vi "Module Loop.vi"(8 "error in (no error)":errorcluster, 11 "Telemetry Command Module in":refnum<class "Telemetry Command Module.lvclass">) -> (0 "error out":errorcluster, 3 "Telemetry Command Module out":refnum<class "Telemetry Command Module.lvclass">)   [LabVIEW 2020, in "VolatusGUI.lvlib" / "Telemetry Command Module.lvclass"]
uses:
  Telemetry Command Module.lvclass
  C:/dev/lv20CE/relink/lv-volatus/Volatus/Module/Module.lvclass
  Volatus/Module/Module.lvclass/Module.ctl
  Volatus/Module/Module.lvclass
  Volatus/MessageQ/MessageQ.lvclass/MessageQ.ctl
  Channel Selection.ctl
  <vilib>/Utility/error.llb/Error Cluster From Error Code.vi
  Telemetry Command Module.lvclass/Telemetry Command Module.ctl
  Volatus/MessageQ/MessageQ.lvclass
panel:
  in  "Clear Filter":bool
  in  "Filter":string
  in  "Tree":string(tree)
  out "error out 2":errorcluster
  out "Resource":string
  out "Group":string
  out "Task":string
  out "Channel":string
  out "Node":string
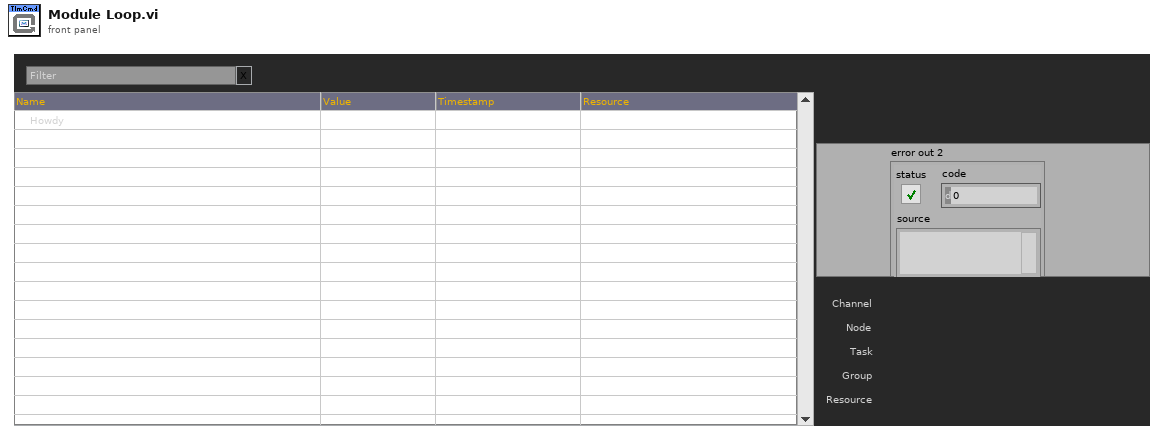
[diagram p1: front panel]
types:
  T1 = typedef "imagedata.ctl" = cluster{"image type":i32, "image depth":i32, "image":u8[], "mask":u8[], "colors":u32[], "Rectangle":cluster{"left":i16, "top":i16, "right":i16, "bottom":i16}}
  T2 = enum32{"Invalid", "Standard", "Closed", "Hidden", "Minimized", "Maximized"}
  T3 = typedef "VolatusGUI.lvlib/Telemetry Command Module.lvclass/Channel Selection.ctl" = cluster{"Node":string, "Group":string, "Channel":string}
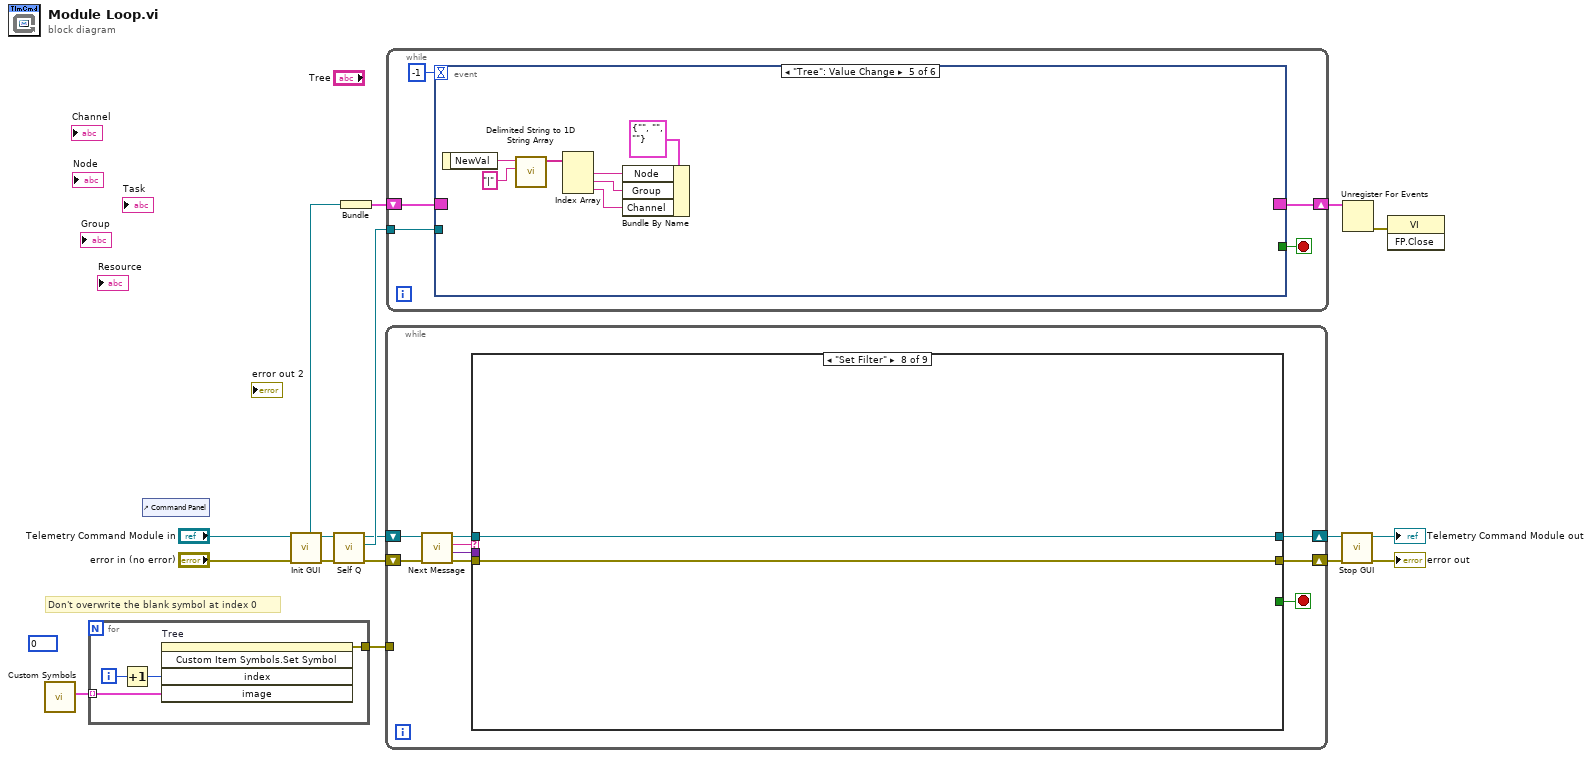
[diagram p0: block diagram]
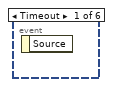
[diagram p2: hidden frame]
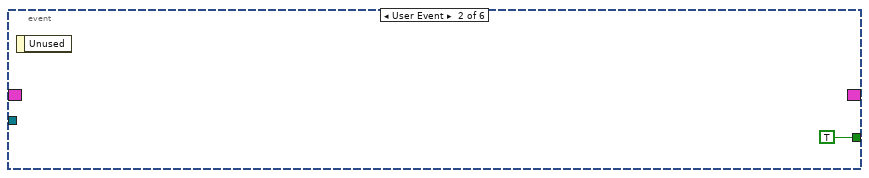
[diagram p3: hidden frame]
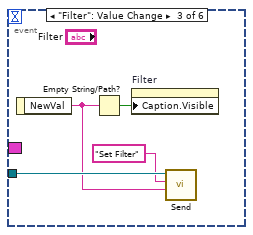
[diagram p4: hidden frame]
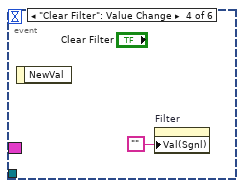
[diagram p5: hidden frame]
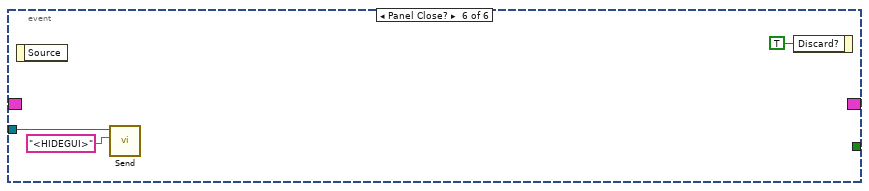
[diagram p6: hidden frame]
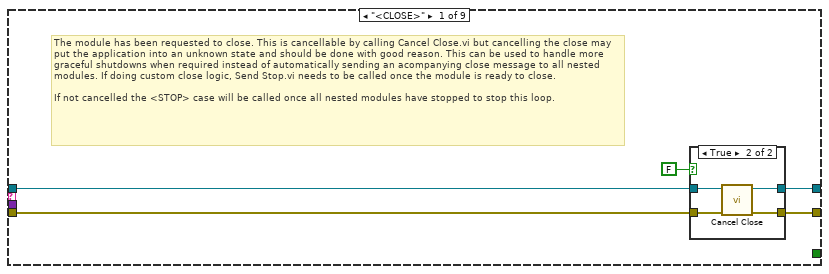
[diagram p7: hidden frame]
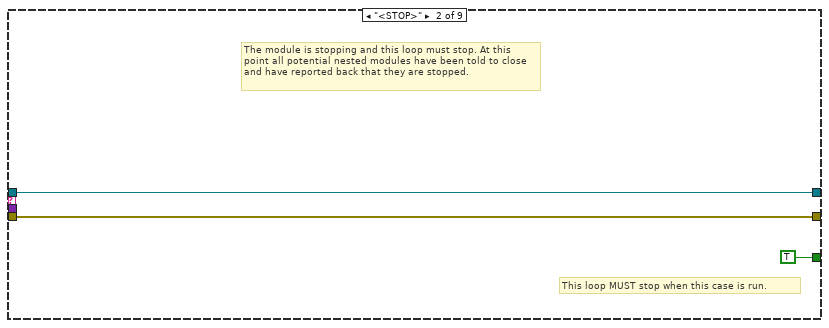
[diagram p9: hidden frame]
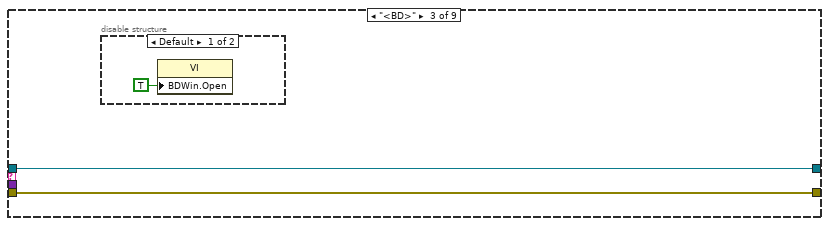
[diagram p10: hidden frame]
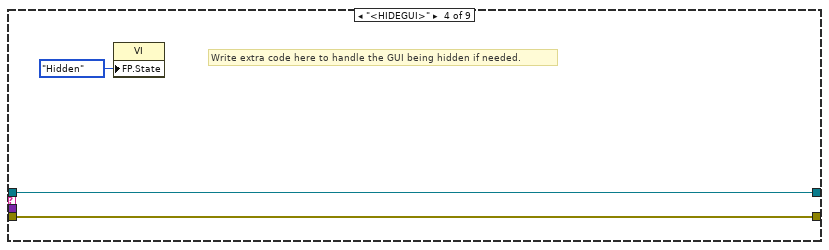
[diagram p12: hidden frame]
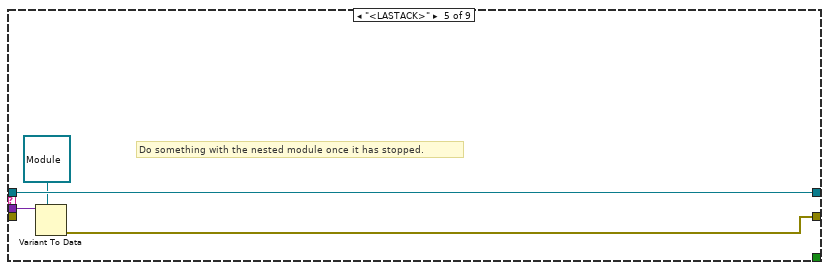
[diagram p13: hidden frame]
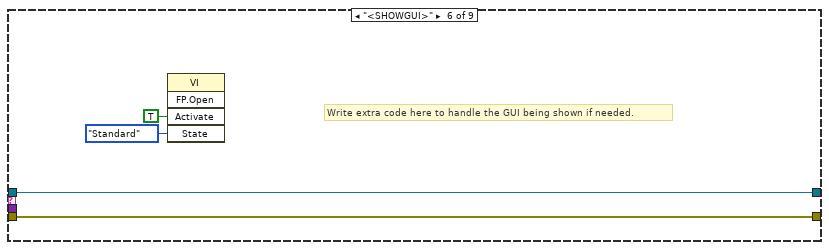
[diagram p14: hidden frame]
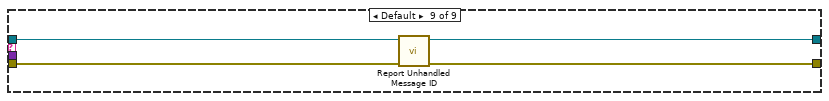
[diagram p16: hidden frame]
diagram:
  (unwired) 0
  # "Don't overwrite the blank symbol at index 0"
  n1 = call "Custom Symbols.vi"() -> ("Custom symbols"=w2:T1[])  [unwired: 11 in]
  n2 = for {
    tunnel: w2 -> [w17] mode=indexing
    tunnel: [w16] -> w1
    i -> [w19]
    n3 = Increment(x=w19) -> (x+1=w18:i32)
    n4 = invoke on="Tree" class="Tree (strict)" method="Custom Item Symbols.Set Symbol"("index"=w18, "image"=w17) -> (error out=w16:errorcluster)  [unwired: 3 in, 4 out]
  }
  n5 = control-ref of="Command Panel"() -> ()  [unwired: 1 out]
  n6 = call "Init GUI.vi"("Module in"="Telemetry Command Module in") -> ("Module out"=w9:refnum<class "Telemetry Command Module.lvclass">, "Event Reg"=w14:refnum<event-registration>)  [unwired: 9 in]
  n7 = call "Self Q.vi"("Module in"=w9) -> ("Self Q"=w8:refnum<class "MessageQ.lvclass">, "Module out"=w7:refnum<class "Telemetry Command Module.lvclass">)  [unwired: 9 in]
  n8 = Bundle("Event Reg"=w14) -> (w10:cluster{"Event Reg":refnum<event-registration>})  [unwired: 1 in]
  n9 = while {
    shift-right: [w23] -> w12
    shift-left: w7 -> [w28]
    shift-right: [w22] -> w13
    shift-left: "error in (no error)" -> [w27]
    tunnel: w1 -> [_]
    stop <- w21 stop-if-true
    n10 = call "Next Message.vi"("error in (no error)"=w27, "Module in"=w28) -> ("error out"=w26:errorcluster, "Data"=w20:variant, "ID"=w25:string, "Module out"=w24:refnum<class "Telemetry Command Module.lvclass">)  [unwired: 6 in]
    n11 = case shown="\"Set Filter\"" w25 {
      tunnel: w26 -> [w31 w41 w43 w47 _ w55 w57 w59 w64]
      tunnel: w24 -> [w32 w42 w44 w48 w52 w56 w58 w60 w62]
      tunnel: [w30 w42 w44 w48 w52 w56 w58 w60 w61] -> w23
      tunnel: [w29 w41 w43 w47 w49 w55 w57 w59 w63] -> w22
      tunnel: [_ TRUE _ _ _ _ _ _ _] -> w21
      tunnel: w20 -> [_ _ _ _ w51 _ _ _ _]
      frame "<CLOSE>" {
        # "The module has been requested to close. This is cancellable by calling Cancel Close.vi but cancelling the close may put the application into an unknown state and should be done with good reason. This can be used to handle more graceful shutdowns when required instead of automatically sending an acompanying close message to all nested modules. If doing custom close logic, Send Stop.vi needs to be called once the module is ready to close.\n\nIf not cancelled the <STOP> case will be called once all nested modules have stopped to stop this loop."
        n12 = case shown="True" FALSE {
          tunnel: w31 -> [w34 w39]
          tunnel: [w34 w38] -> w29
          tunnel: w32 -> [w35 w37]
          tunnel: [w35 w36] -> w30
          frame False {
          }
          frame True {
            n13 = call "Cancel Close.vi"("error in (no error)"=w39, "Module in"=w37) -> ("error out"=w38:errorcluster, "Module out"=w36:refnum<class "Telemetry Command Module.lvclass">)  [unwired: 8 in]
          }
        }
      }
      frame "<STOP>" {
        # "This loop MUST stop when this case is run."
        # "The module is stopping and this loop must stop. At this point all potential nested modules have been told to close and have reported back that they are stopped."
      }
      frame "<BD>" {
        n14 = disable-structure shown="Default" {
          frame condition #0 (active) {
            n15 = property class="VI"("BDWin.Open"=TRUE ("Block Diagram Window:Open")) -> ()  [unwired: 2 in, 2 out]
          }
          frame condition #1 {
          }
        }
      }
      frame "<HIDEGUI>" {
        # "Write extra code here to handle the GUI being hidden if needed."
        n16 = property class="VI"("FP.State"=T2."Hidden" ("Front Panel Window:State")) -> ()  [unwired: 2 in, 2 out]
      }
      frame "<LASTACK>" {
        # "Do something with the nested module once it has stopped."
        n17 = Variant To Data(type=refnum<class "Module.lvclass"> refnum ("Volatus:Module"), Variant=w51) -> (error out=w49:errorcluster)  [unwired: 1 in, 1 out]
      }
      frame "<SHOWGUI>" {
        # "Write extra code here to handle the GUI being shown if needed."
        n18 = invoke class="VI" method="FP.Open"("Activate"=TRUE ("Activate?"), "State"=T2."Standard") -> ()  [unwired: 3 in, 5 out]
      }
      frame "<TIMEOUT>" {
        # "No message for this module was received in time"
      }
      frame "Set Filter" {
      }
      frame Default {
        n19 = call "Report Unhandled Message ID.vi"("error in (no error)"=w64, "Module in"=w62) -> ("error out"=w63:errorcluster, "Module out"=w61:refnum<class "Telemetry Command Module.lvclass">)  [unwired: 8 in]
      }
    }
  }
  n20 = while {
    tunnel: w8 -> [w69]
    shift-right: [w67] -> w11
    shift-left: w10 -> [w68]
    stop <- w66 stop-if-true
    n21 = event shown="[4] \"Tree\": Value Change" {
      selector: w68 -> [_ _ _ _ _ _]
      dyn-events: [_ _ _ _ _ _] -> w67
      timeout: -1 -> [_ _ _ _ _ _]
      tunnel: w69 -> [_ _ w74 _ _ w84]
      tunnel: [_ TRUE _ _ _ _] -> w66
      event Timeout {
        n22 = event-data() -> ()  [unwired: 1 in, 1 out]
      }
      event User Event {
        n23 = event-data() -> ()  [unwired: 1 in, 1 out]
      }
      event "Filter": Value Change {
        n24 = event-data() -> ("NewVal"=w73:string)  [unwired: 1 in]
        n25 = Empty String/Path?(string/path=w73) -> (empty?=w71:bool)
        n26 = property on="Filter" class="Str"("Caption.Visible"=w71) -> ()  [unwired: 2 in, 2 out]
        n27 = call "Send.vi"("Data"=w73, "ID"="Set Filter", "MessageQ in"=w74) -> ()  [unwired: 7 in, 2 out]
      }
      event "Clear Filter": Value Change {
        n28 = event-data() -> ()  [unwired: 1 in, 1 out]
        n29 = property on="Filter" class="Str"("Val(Sgnl)"="") -> ()  [unwired: 2 in, 2 out]
      }
      event "Tree": Value Change {
        n30 = event-data() -> ("NewVal"=w82:string)  [unwired: 1 in]
        n31 = call <vilib>:"Delimited String to 1D String Array.vi"("delimiter"="|", "delimited string"=w82) -> ("string array"=w80:string[])  [unwired: 9 in]
        n32 = Index Array(array=w80) -> (element #1=w78:string, element #2=w77:string, element #3=w76:string)  [unwired: 3 in]
        n33 = Bundle By Name(cluster=T3 {"Node"="", "Group"="", "Channel"=""} ("Channel Selection"), "Node"=w78, "Group"=w77, "Channel"=w76) -> ()  [unwired: 1 out]
      }
      event Panel Close? {
        n34 = event-data() -> ()  [unwired: 1 in, 1 out]
        n35 = call "Send.vi"("ID"="<HIDEGUI>", "MessageQ in"=w84) -> ()  [unwired: 8 in, 2 out]
        n36 = event-data("Discard?"=TRUE) -> ()  [unwired: 1 in, 1 out]
      }
    }
  }
  n37 = call "Stop GUI.vi"("error in (no error)"=w13, "Module in"=w12) -> ("error out"=→"error out":errorcluster, "Module out"=→"Telemetry Command Module out":refnum<class "Telemetry Command Module.lvclass">)  [unwired: 8 in]
  n38 = Unregister For Events(event registration refnum=w11) -> (error out=w15:errorcluster)  [unwired: 1 in]
  n39 = invoke class="VI" method="FP.Close"(error in=w15) -> ()  [unwired: 2 in, 3 out]
